vi "configRead.vi"(9 "refDes":string, 10 "Self":T2={"refDes"="ERR000", "IP"="localhost", "DI"=0, "DO"=0, "AI"=0, "AO"=0, "Description"="ERR", "TC"=0, "channelDefinitions"=[]}, 11 "configPath":path=path "C:/Users/miles/OneDrive - Embry-Riddle Aeronautical University/Admin/Facilities/TC3/TC3 DAC/Code/Sandbox/Node based/controlNode/Configuration/nodeConfig_0.xlsx") -> (2 "Self":T2={"refDes"="ERR000", "IP"="localhost", "DI"=0, "DO"=0, "AI"=0, "AO"=0, "Description"="ERR", "TC"=0, "channelDefinitions"=[]}, 3 "Cancel/Err":bool)   [LabVIEW 2024]
uses:
  controls/self.ctl
  controls/channelDefinition.ctl
  controls/dataRefs.ctl
panel:
  in  "dataRef":T1
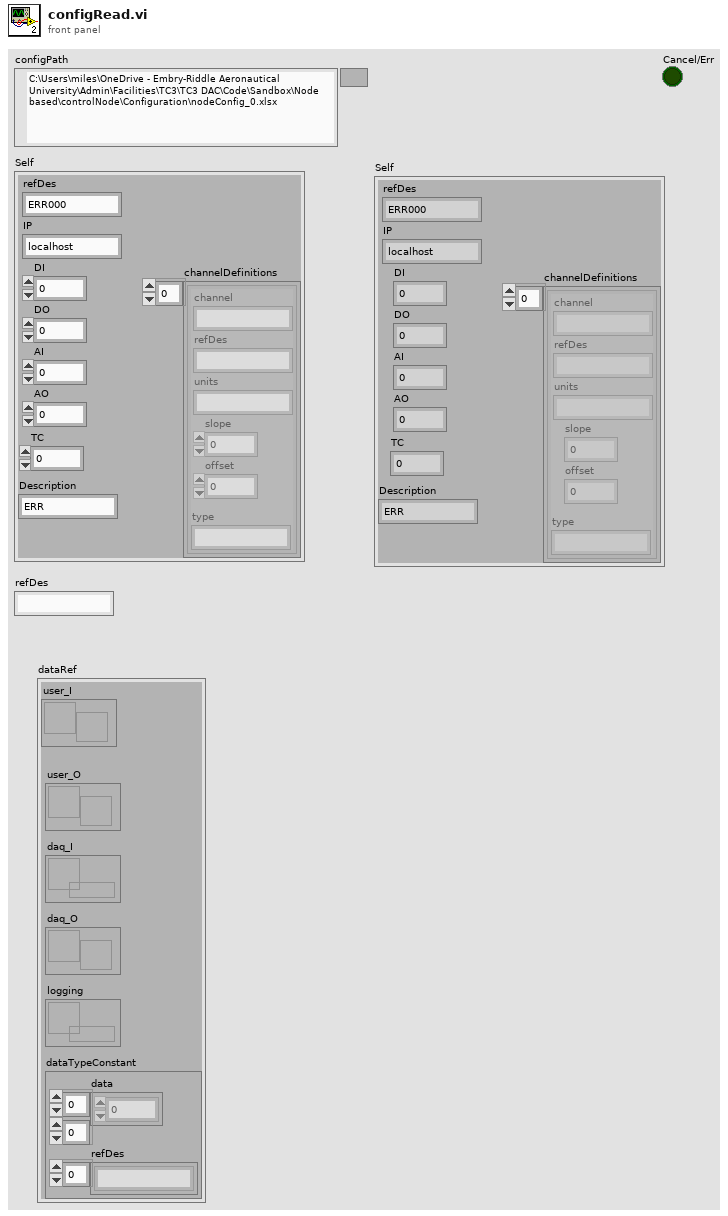
[diagram p1: front panel]
types:
  T1 = typedef "dataRefs.ctl" = cluster{"dataTypeConstant":cluster{"data":dbl[][], "refDes":string[]}, "user_I":refnum<notifier>, "user_O":refnum<notifier>, "daq_O":refnum<notifier>, "logging":refnum<queue>, "daq_I":refnum<queue>}
  T2 = typedef "self.ctl" = cluster{"refDes":string, "IP":string, "DI":i32, "DO":i32, "AI":i32, "AO":i32, "Description":string, "TC":i32, "channelDefinitions":T3[]}
  T3 = typedef "channelDefinition.ctl" = cluster{"channel":string, "refDes":string, "units":string, "slope":dbl, "offset":dbl, "type":string}
  T4 = cluster{"[0]":string, "[1]":string, "[2]":string, "[3]":string, "[4]":string, "[5]":string, "[6]":string, "[7]":string, "[8]":string}
  T5 = cluster{"[0]":i32, "[1]":i32, "[2]":i32, "[3]":i32, "[4]":i32, "[5]":i32, "[6]":i32, "[7]":i32, "[8]":i32}
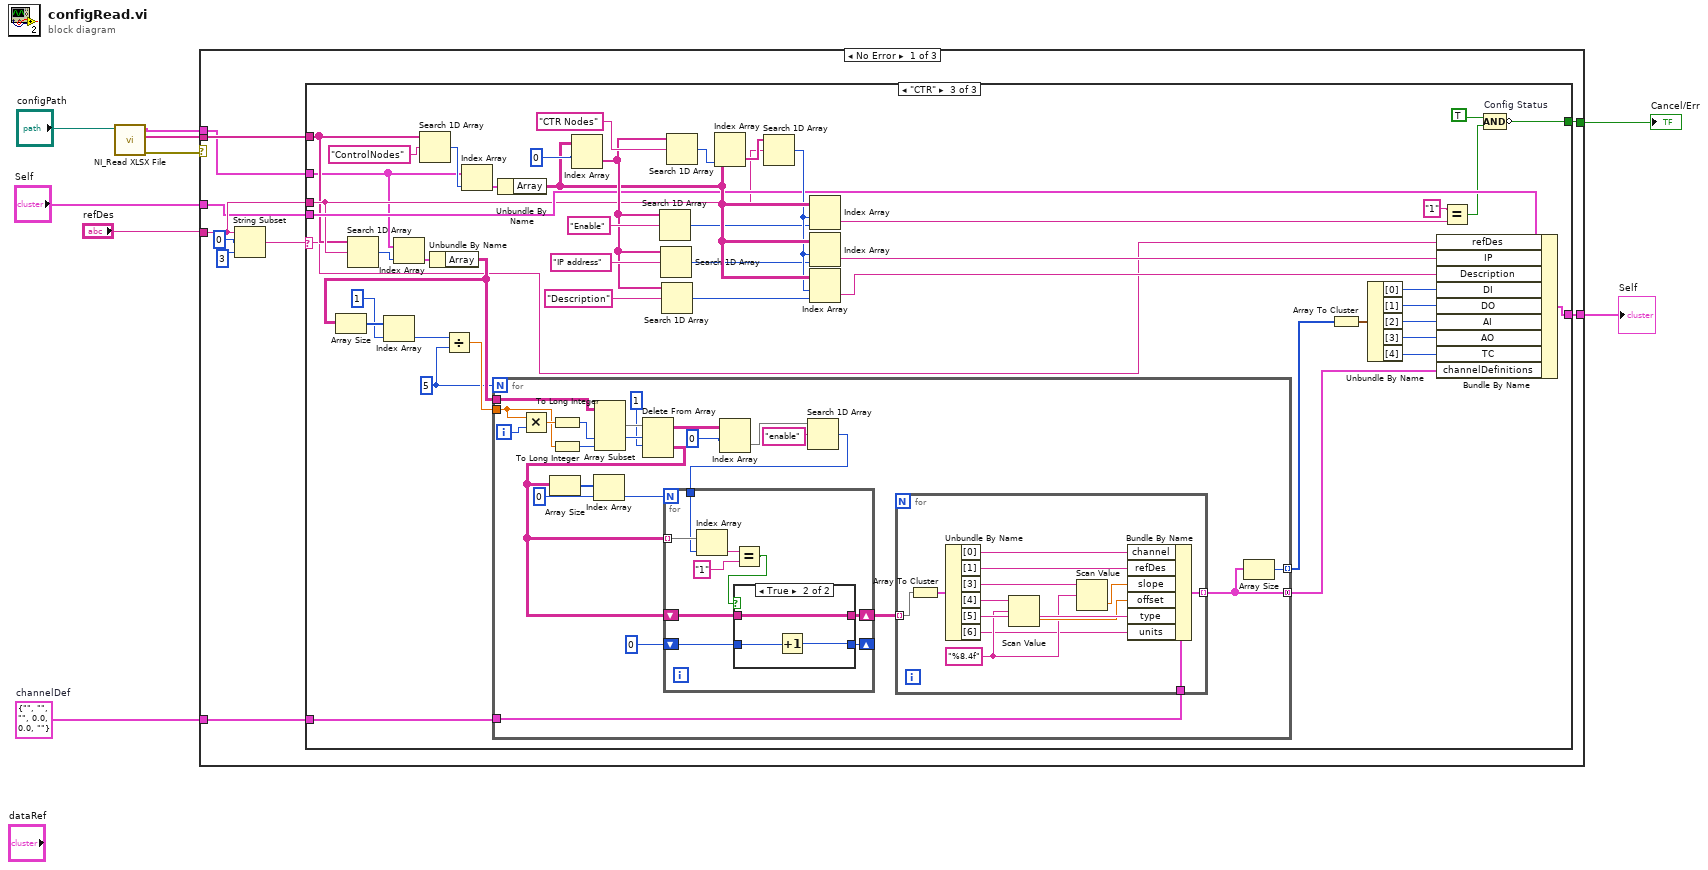
[diagram p0: block diagram]
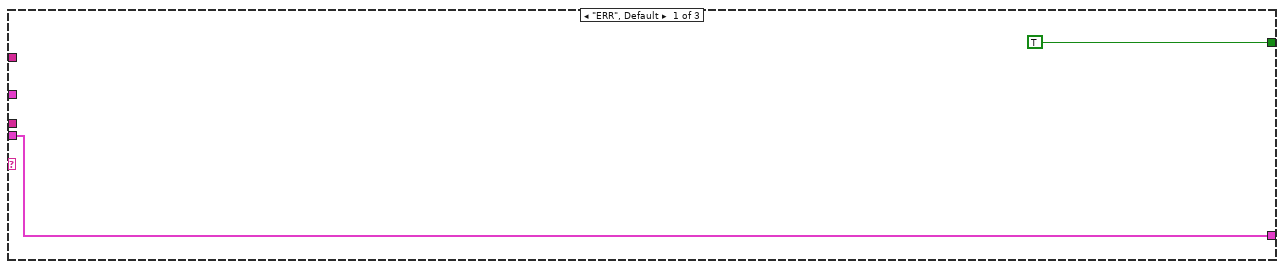
[diagram p2: hidden frame]
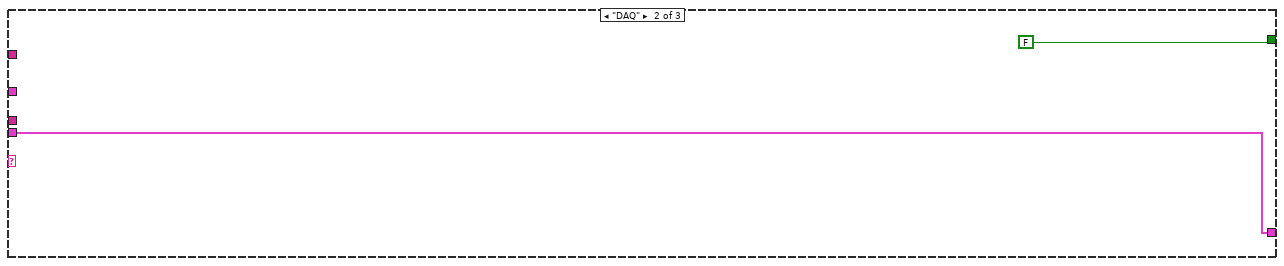
[diagram p3: hidden frame]
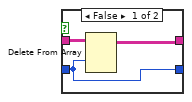
[diagram p4: hidden frame]
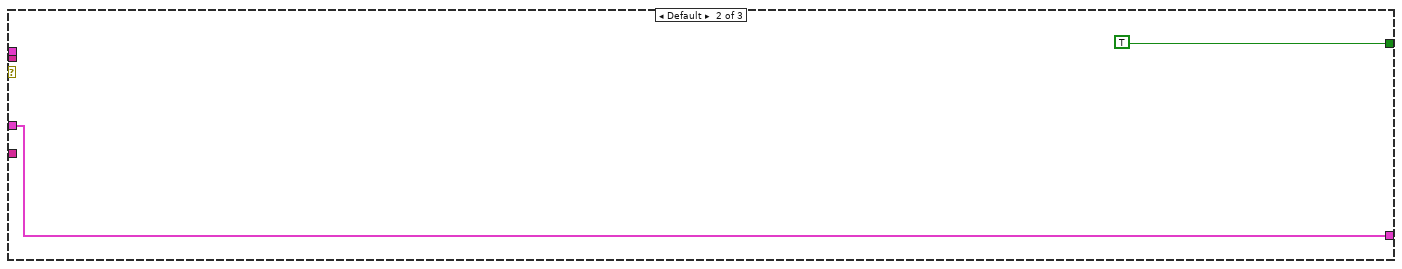
[diagram p5: hidden frame]
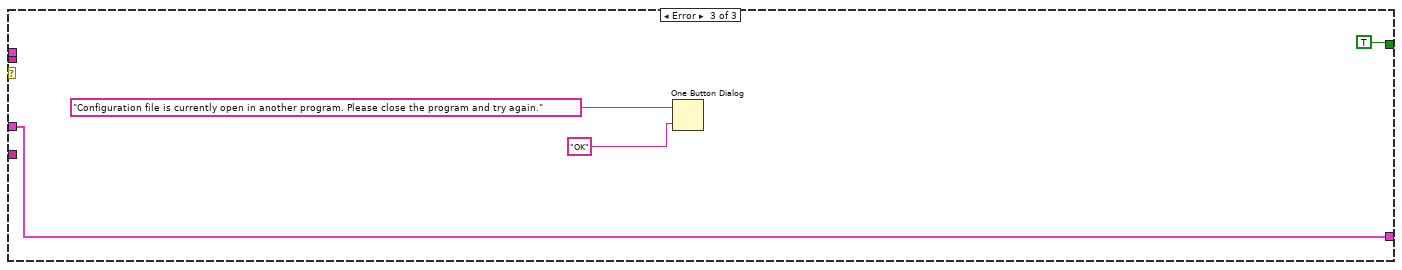
[diagram p6: hidden frame]
diagram:
  w2 = T3 {"channel"="", "refDes"="", "units"="", "slope"=0.0, "offset"=0.0, "type"=""}  # channelDef
  n1 = call "NI_Read XLSX File.vi"("XLSX File"="configPath") -> ("error out"=w8:errorcluster, "Sheet Names"=w7:string[], "Sheet Data"=w6:cluster{"Array":string[][]}[])  [unwired: 8 in]
  n2 = case shown="No Error" w8 {
    tunnel: [w13 TRUE TRUE] -> w9
    tunnel: w7 -> [w16 _ _]
    tunnel: w6 -> [w15 _ _]
    tunnel: "refDes" -> [w14 _ _]
    tunnel: "Self" -> [w12 w120 w124]
    tunnel: [w11 w120 w124] -> w3
    tunnel: w2 -> [w10 _ _]
    frame No Error {
      n3 = String Subset(string=w14, offset (0)=0, length (rest)=3 ("length (rest)")) -> (substring=w17:string)
      n4 = case shown="\"CTR\"" w17 {
        selector: w17 -> [_ _ w24]
        tunnel: w16 -> [_ _ w41]
        tunnel: w15 -> [_ _ w40]
        tunnel: w14 -> [_ _ w42]
        tunnel: [TRUE FALSE w61] -> w13
        tunnel: w12 -> [w20 w22 w51]
        tunnel: [w20 w22 w48] -> w11
        tunnel: w10 -> [_ _ w34]
        frame "ERR", Default {
        }
        frame "DAQ" {
        }
        frame "CTR" {
          w35 = 5 ("y")
          n5 = Search 1D Array(1D array=w41, element=w42) -> (index of element=w44:i32)  [unwired: 1 in]
          n6 = Index Array(array=w40, index=w44) -> (element=w43:cluster{"Array":string[][]})
          n7 = Search 1D Array(1D array=w41, element="ControlNodes") -> (index of element=w68:i32)  [unwired: 1 in]
          n8 = Unbundle By Name(w43) -> ("Array"=w39:string[][])
          n9 = Array Size(array=w39) -> (size(s)=w38:i32[])
          n10 = Index Array(array=w38, index=1) -> (element=w25:i32)
          n11 = Divide(x=w25, y=w35) -> (x/y=w36:dbl)
          n12 = Index Array(array=w40, index=w68) -> (element=w67:cluster{"Array":string[][]})
          n13 = for {
            N: w35 -> [_]
            tunnel: w39 -> [w91]
            tunnel: w36 -> [w89]
            tunnel: w34 -> [w79]
            tunnel: [w78] -> w26 mode=concatenating
            tunnel: [w77] -> w33 mode=indexing
            i -> [w76]
            n14 = Multiply(x=w89, y=w76) -> (x*y=w90:dbl)
            n15 = To Long Integer(number=w90) -> (32bit integer=w88:i32)
            n16 = To Long Integer(number=w89) -> (32bit integer=w86:i32)
            n17 = Array Subset(array=w91, index (col)=w88, length (col)=w86) -> (w87:string[][])  [unwired: 2 in]
            n18 = Delete From Array(array=w87, length=w86, index (row)=1) -> (deleted portion=w81:string[][], array with subset deleted=w72:string[][])  [unwired: 1 in]
            n19 = Array Size(array=w81) -> (size(s)=w85:i32[])
            n20 = Index Array(array=w85, index=0) -> (element=w83:i32)
            n21 = Index Array(array=w72, index (row)=0) -> (element=w74:string[])  [unwired: 1 in]
            n22 = Search 1D Array(1D array=w74, element="enable") -> (index of element=w71:i32)  [unwired: 1 in]
            n23 = for {
              N: w83 -> [_]
              tunnel: w81 -> [w111] mode=indexing
              shift-right: [w108] -> w80
              shift-left: w81 -> [w110]
              tunnel: w71 -> [w107]
              shift-right: [w105] -> _
              shift-left: 0 -> [w106]
              n24 = Index Array(array=w111, index=w107) -> (element=w113:string)
              n25 = Equal?(x=w113, y="1") -> (x = y?=w109:bool)
              n26 = case shown="True" w109 {
                tunnel: w110 -> [w116 w119]
                tunnel: [w115 w119] -> w108
                tunnel: w106 -> [w114 w118]
                tunnel: [w114 w117] -> w105
                frame False {
                  n27 = Delete From Array(array=w116, index (row)=w114) -> (array with subset deleted=w115:string[][])  [unwired: 2 in, 1 out]
                }
                frame True {
                  n28 = Increment(x=w118) -> (x+1=w117:i32)
                }
              }
            }
            n29 = for {
              tunnel: w80 -> [w95] mode=indexing
              tunnel: w79 -> [w94]
              tunnel: [w93] -> w78 mode=indexing
              w96 = "%8.4f"
              n30 = Array To Cluster(array=w95) -> (cluster=w104:T4)
              n31 = Unbundle By Name(w104) -> ("[0]"=w103:string, "[1]"=w102:string, "[3]"=w100:string, "[4]"=w98:string, "[5]"=w101:string, "[6]"=w92:string)
              n32 = Scan Value(string=w98, format string=w96) -> (value=w97:dbl)  [unwired: 1 in, 1 out]
              n33 = Scan Value(string=w100, format string=w96) -> (value=w99:dbl)  [unwired: 1 in, 1 out]
              n34 = Bundle By Name(cluster=w94, "channel"=w103, "refDes"=w102, "slope"=w99, "offset"=w97, "type"=w101, "units"=w92) -> (w93:T3)
            }
            n35 = Array Size(array=w78) -> (size(s)=w77:i32)
          }
          n36 = Unbundle By Name(w67) -> ("Array"=w56:string[][])
          n37 = Index Array(array=w56, index (row)=0) -> (element=w57:string[])  [unwired: 1 in]
          n38 = Search 1D Array(1D array=w57, element="Enable") -> (index of element=w54:i32)  [unwired: 1 in]
          n39 = Search 1D Array(1D array=w57, element="IP address") -> (index of element=w53:i32)  [unwired: 1 in]
          n40 = Search 1D Array(1D array=w57, element="Description") -> (index of element=w52:i32)  [unwired: 1 in]
          n41 = Search 1D Array(1D array=w57, element="CTR Nodes") -> (index of element=w64:i32)  [unwired: 1 in]
          n42 = Index Array(array=w56, index (col)=w64) -> (element=w63:string[])  [unwired: 1 in]
          n43 = Search 1D Array(1D array=w63, element=w42) -> (index of element=w55:i32)  [unwired: 1 in]
          n44 = Index Array(array=w56, index (row)=w55, index (col)=w54) -> (element=w46:string)
          n45 = Index Array(array=w56, index (row)=w55, index (col)=w53) -> (element=w50:string)
          n46 = Index Array(array=w56, index (row)=w55, index (col)=w52) -> (element=w49:string)
          n47 = Array To Cluster(array=w33) -> (cluster=w32:T5)
          n48 = Unbundle By Name(w32) -> ("[0]"=w31:i32, "[1]"=w30:i32, "[2]"=w29:i32, "[3]"=w28:i32, "[4]"=w27:i32)
          n49 = Bundle By Name(cluster=w51, "refDes"=w24, "IP"=w50, "Description"=w49, "DI"=w31, "DO"=w30, "AI"=w29, "AO"=w28, "TC"=w27, "channelDefinitions"=w26) -> (w48:T2)
          n50 = Equal?(x="1", y=w46) -> (x = y?=w45:bool)
          n51 = Compound Arithmetic op=AND "Config Status"(TRUE, w45) -> (invert w61:bool)
        }
      }
    }
    frame Default {
    }
    frame Error {
      n52 = One Button Dialog(message="Configuration file is currently open in another program. Please close the program and try again.", button name ("OK")="OK") -> ()  [unwired: 1 out]
    }
  }
  "Cancel/Err" <- w9
  "Self" <- w3
